vi "p6100_read_setpoint.vi"(0 "VISA in":refnum<visa-resource-name>, 1 "Serial Parameters":T1, 2 "Setpoint":cluster{dbl, dbl}, 3 "error in":errorcluster) -> (5 "VISA out":refnum<visa-resource-name>, 6 "Temp":cluster{"Bottom":dbl, "Top":dbl}, 7 "error out":errorcluster)   [LabVIEW 2011]
uses:
  <vilib>/NI Modbus.llb/MB Serial Master Query Read Input Registers (poly).vi
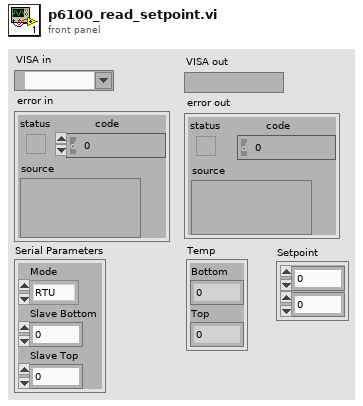
[diagram p1: front panel]
types:
  T1 = cluster{"Mode":enum16{"RTU", "ASCII"}, "Slave Bottom":u8, "Slave Top":u8}
  T2 = cluster{"Mode":enum16{"RTU", "ASCII"}, "Slave Bottom":u8}
  T3 = cluster{"Mode":enum16{"RTU", "ASCII"}, "Slave Top":u8}
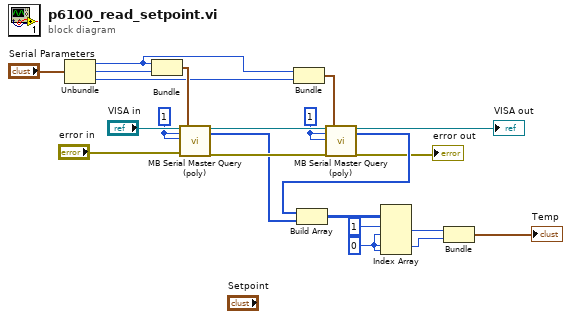
[diagram p0: block diagram]
diagram:
  w4 = 0 ("disabled index (col)")
  w17 = u16 1 ("Quantity")
  w18 = u16 1 ("Starting Address")
  n1 = Unbundle("Serial Parameters") -> ("Mode"=w11:enum16{"RTU", "ASCII"}, "Slave Bottom"=w15:u8, "Slave Top"=w13:u8)
  n2 = Bundle("Mode"=w11, "Slave Bottom"=w15) -> (w14:T2)  [unwired: 1 in]
  n3 = call-poly <vilib>:"MB Serial Master Query (poly).vi"("VISA resource name"="VISA in", "Starting Address"=w18, "Quantity"=w18, "error in"="error in", "Serial Parameters"=w14) -> ("VISA resource name out"=w22:refnum<visa-resource-name>, "Input Registers"=w10:u16[], "error out"=w21:errorcluster)  [unwired: 11 in, 1 out]
  n4 = Bundle("Mode"=w11, "Slave Top"=w13) -> (w12:T3)  [unwired: 1 in]
  n5 = call-poly <vilib>:"MB Serial Master Query (poly).vi"("VISA resource name"=w22, "Starting Address"=w17, "Quantity"=w17, "error in"=w21, "Serial Parameters"=w12) -> ("VISA resource name out"=→"VISA out":refnum<visa-resource-name>, "Input Registers"=w9:u16[], "error out"=→"error out":errorcluster)  [unwired: 11 in, 1 out]
  n6 = Build Array(w9, w10) -> (w8:u16[][])
  n7 = Index Array(array=w8, index (row) #1=1 ("disabled index (col)"), index (col) #1=w4, index (row) #2=w4, index (col) #2=w4) -> (element #1=w7:u16, element #2=w6:u16)
  n8 = Bundle("Numeric"=w7, "Numeric"=w6) -> (→"Temp":cluster{"Numeric":u16, "Numeric":u16})  [unwired: 1 in]
